vi "create1.vi"(9 "center":i32, 10 "X size":i32, 11 "max Y size":i32) -> (2 "size":i32, 3 "Array":i32[][](array[numeric]))   [LabVIEW 2020]
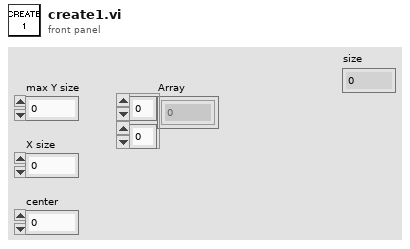
[diagram p1: front panel]
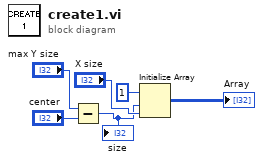
[diagram p0: block diagram]
diagram:
  n1 = Subtract(x="max Y size", y="center") -> (x-y=w2:i32)
  "size" <- w2
  n2 = Initialize Array(1, w2, "X size") -> (→"Array":i32[][])
